vi "Stop Fan.vi"(8 "error in (no error)":errorcluster, 11 "Fan Controller Ref":refnum<data-value>) -> (0 "error out":errorcluster, 3 "Fan Controller Ref out":refnum<data-value>)   [LabVIEW 2019, in "Fan Controller Ref.lvclass"]
uses:
  <vilib>/gpm_packages/@cs/Car-wash/Source/Fan Controller Ref/Fan Controller Ref.lvclass
  <vilib>/gpm_packages/@cs/Car-wash/Source/iFan Controller/iFan Controller.lvclass
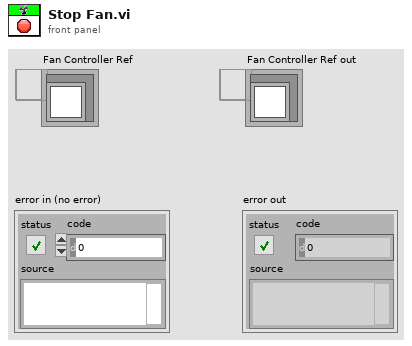
[diagram p1: front panel]
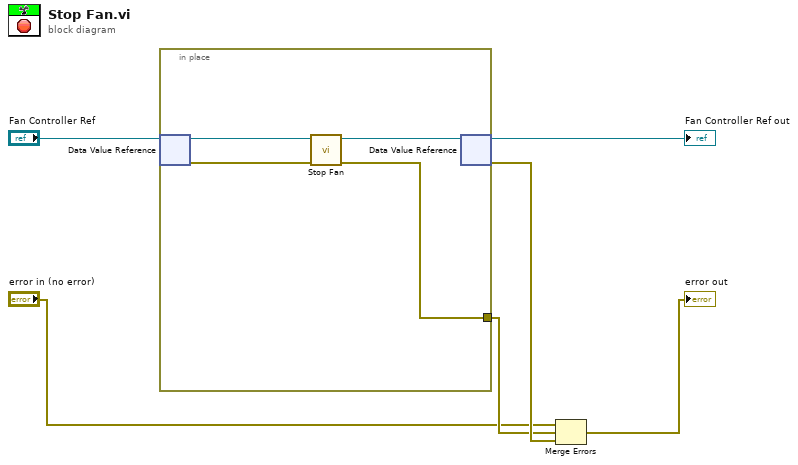
[diagram p0: block diagram]
diagram:
  n1 = in-place {
    in-place-border: [w7] -> w5
    n2 = in-place-dvr #1("Fan Controller Ref") -> (w10:refnum<class "iFan Controller.lvclass">, w8:errorcluster)
    n3 = call-dynamic "Stop Fan.vi"("error in (no error)"=w8, "iFan Controller in"=w10) -> ("error out"=w7:errorcluster, "iFan Controller out"=w9:refnum<class "iFan Controller.lvclass">)  [unwired: 8 in]
    n4 = in-place-dvr #1(w9) -> (→"Fan Controller Ref out":refnum<data-value>, w6:errorcluster)
  }
  n5 = Merge Errors("error in (no error)", w5, w6) -> (→"error out":errorcluster)
